vi "Create_DO_WF.vi"(8 "error in":errorcluster) -> (0 "error out":errorcluster)   [LabVIEW 2025]
panel:
  out "Samples":u32
  out "Digital waveform 2":digitalwaveform[](graph)
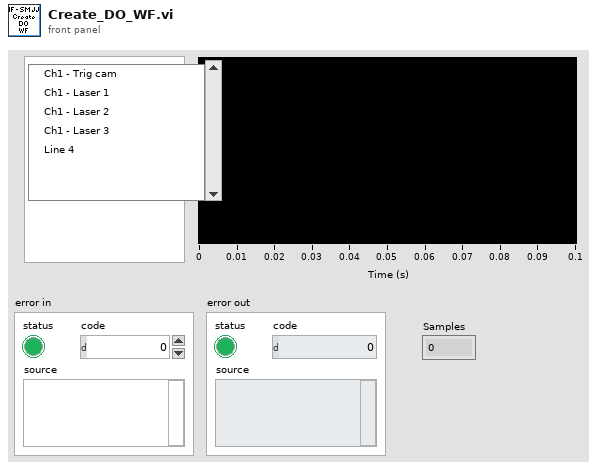
[diagram p1: front panel]
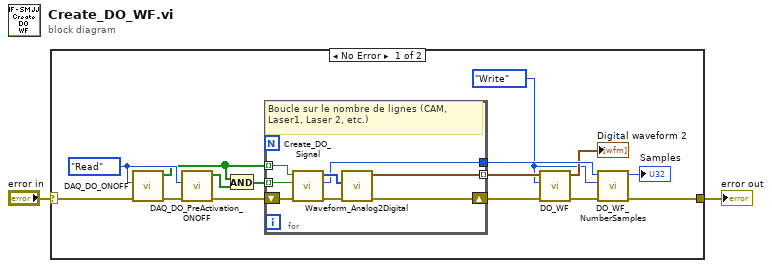
[diagram p0: block diagram]
diagram:
  n1 = case shown="No Error" "error in" {
    selector: "error in" -> [w17 w26]
    tunnel: [w14 w26] -> w1
    frame No Error {
      w8 = enum16{"Write", "Read"}."Read" ("Action")
      w9 = enum16{"Write", "Read"}."Write" ("Action")
      n2 = call "DAQ_DO_ONOFF.vi"("error in"=w17, "Action"=w8) -> ("error out"=w7:errorcluster, "DO | ON/OFF"=w5:bool[])  [unwired: 8 in]
      n3 = call "DAQ_DO_PreActivation_ONOFF.vi"("error in"=w7, "Action"=w8) -> ("error out"=w6:errorcluster, "DO | PreActivation ON/OFF"=w4:bool[])  [unwired: 8 in]
      n4 = And(x=w5, y=w4) -> (x .and. y?=w3:bool[])
      n5 = for {
        tunnel: [w21] -> w13 mode=indexing
        shift-right: [w23] -> w12
        shift-left: w6 -> [w25]
        tunnel: [w20] -> w16
        tunnel: w5 -> [w19] mode=indexing
        tunnel: w3 -> [w18] mode=indexing
        # "Boucle sur le nombre de lignes (CAM, Laser1, Laser 2, etc.)"
        n6 = call "Create_DO_Signal.vi"("error in"=w25, "Pre-Activation?"=w18, "On/Off"=w19) -> ("error out"=w24:errorcluster, "Samples"=w20:u32, "WF"=w22:u8[])  [unwired: 6 in]
        n7 = call "Waveform_Analog2Digital.vi"("error in (no error)"=w24, "\"Binary waveform\""=w22) -> ("error out"=w23:errorcluster, "Digital signal"=w21:digitalwaveform)  [unwired: 8 in]
      }
      n8 = call "DO_WF.vi"("error in"=w12, "Action"=w9, "Digital WF"=w13) -> ("error out"=w11:errorcluster, "Digital WF"=→"Digital waveform 2":digitalwaveform[])  [unwired: 7 in]
      n9 = call "DO_WF_NumberSamples.vi"("error in"=w11, "Action"=w9, "DO_WF_NumberOfSamples"=w16) -> ("error out"=w14:errorcluster, "DO_WF_NumberOfSamples"=→"Samples":u32)  [unwired: 7 in]
    }
    frame Error {
    }
  }
  "error out" <- w1
